vi "Accelration Control (by Throttle).vi"(1 "reinitialize? (F)":bool, 2 "acc":dbl, 3 "input":dbl) -> (0 "output":dbl format="%.2f")   [LabVIEW 2011]
uses:
  <vilib>/addons/control/pid/pid.llb/PID Lead-Lag (DBL).vi
  <vilib>/addons/control/pid/NI_PID_pid.lvlib
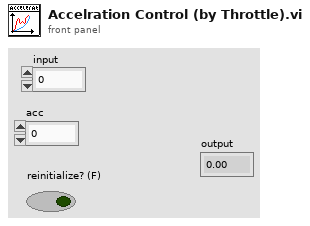
[diagram p1: front panel]
types:
  T1 = cluster{"gain":dbl, "lag time (min)":dbl, "lead time (min)":dbl}
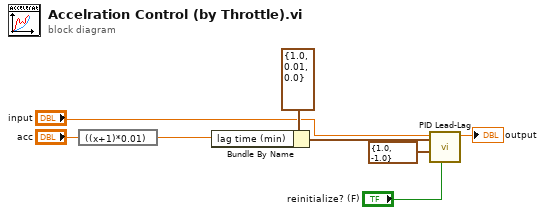
[diagram p0: block diagram]
diagram:
  n1 = expression code="((x+1)*0.01)"("acc") -> (w6:dbl)
  n2 = Bundle By Name(cluster=T1 {"gain"=1.0, "lag time (min)"=0.01, "lead time (min)"=0.0} ("tuning parameters"), "lag time (min)"=w6) -> (w5:T1)
  n3 = call-poly <vilib>:"PID Lead-Lag.vi"("reinitialize? (F)"="reinitialize? (F)", "output range"=cluster{"output high":dbl, "output low":dbl} {"output high"=1.0, "output low"=-1.0}, "tuning parameters"=w5, "input"="input") -> ("output"=→"output":dbl)  [unwired: 2 in, 3 out]
